vi "Test FFT time2.vi"() -> ()   [LabVIEW 2018]
uses:
  General/type defines/FFT parameters.ctl
  <vilib>/Analysis/4window.llb/windowTd.ctl
  <vilib>/Analysis/NI_AALPro.lvlib
panel:
  out "Waveform Chart":sgl[](graph)
  in  "error in (no error)":errorcluster
  out "time for FFT":dbl
  in  "FFT parameters":T1={"window"=1, "view"={"dB On (F)"=FALSE, "unwrap phase (F)"=FALSE, "convert to degree (F)"=FALSE}, "#A-lines"=1200, "start pixel"=0, "#pixels to save"=300} {"window" items=["Rectangle"=0, "Hanning"=1, "Hamming"=2, "Blackman-Harris"=3, "Exact Blackman"=4, "Blackman"=5, "Flat Top"=6, "4 Term B-Harris "=7, "7 Term B-Harris"=8, "Low Sidelobe"=9, "Blackman Nuttall"=11, "Triangle"=30, "Bartlett-Hanning"=31, "Bohman"=32, "Parzen"=33, "Welch"=34, "Kaiser"=60, "Dolph-Chebyshev"=61, "Gaussian"=62]}
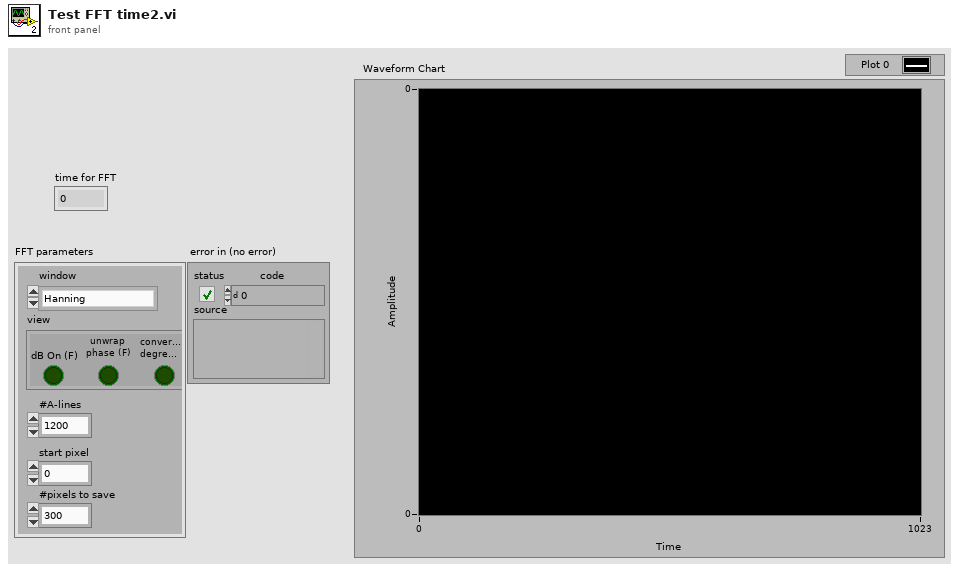
[diagram p1: front panel]
types:
  T1 = typedef "FFT parameters.ctl" = cluster{"window":T2, "view":cluster{"dB On (F)":bool, "unwrap phase (F)":bool, "convert to degree (F)":bool}, "#A-lines":i32, "start pixel":i32, "#pixels to save":i32}
  T2 = typedef "NI_AALPro.lvlib/windowTd.ctl" = u32
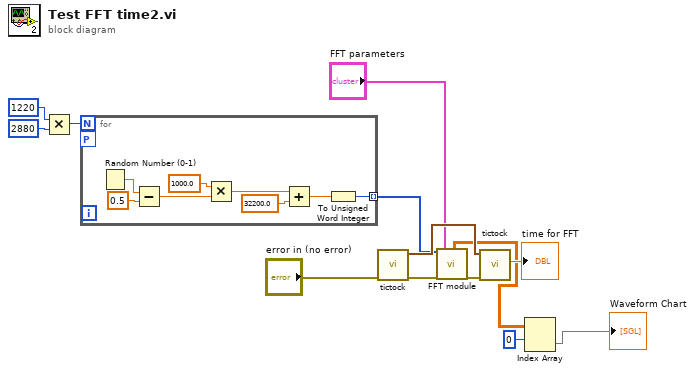
[diagram p0: block diagram]
diagram:
  n1 = Multiply(x=1220, y=2880) -> (x*y=w8:i32)
  n2 = for {
    N: w8 -> [_]
    tunnel: [w21] -> w4 mode=indexing
    workers-P: _ -> [_]
    n3 = Random Number (0-1)() -> (number: 0 to 1=w19:dbl)
    n4 = Subtract(x=w19, y=0.5) -> (x-y=w17:dbl)
    n5 = Multiply(x=1000.0, y=w17) -> (x*y=w15:dbl)
    n6 = Add(x=w15, y=32200.0) -> (x+y=w16:dbl)
    n7 = To Unsigned Word Integer(number=w16) -> (unsigned 16bit integer=w21:u16)
  }
  n8 = call "tictock.vi"("error in (no error)"="error in (no error)") -> ("error out"=w6:errorcluster, "seconds since 1Jan1904"=w11:timestamp)  [unwired: 8 in, 1 out]
  n9 = call "FFT module.vi"("Buffer in"=w4, "error in"=w6, "FFT parameters"="FFT parameters") -> ("Mag A for display"=w1:sgl[][], "error out"=w5:errorcluster)  [unwired: 8 in, 7 out]
  n10 = call "tictock.vi"("error in (no error)"=w5, "seconds since 1Jan1904 2"=w11) -> ("Numeric"=→"time for FFT":dbl)  [unwired: 7 in, 2 out]
  n11 = Index Array(array=w1, index (row)=0) -> (element=→"Waveform Chart":sgl[])  [unwired: 1 in]
